vi "Top_Level_Move_Traverse.vi"(10 "Position":dbl[](array[numeric])=[0.0, 0.0, 0.0] format="%.2f", 11 "Mode":T1) -> (0 "Error String":string, 3 "Trav Position achieved":dbl[](array[numeric]) format="%.2f")   [LabVIEW 2012]
uses:
  Anemometry Sub Vis/Gen Trav/Trav_mode.ctl
  Anemometry Sub Vis/Controls/User_Specific_mode.ctl
  Anemometry Sub Vis/Globals/Trav_pos_global.vi
panel:
  out "Model       Roll      Pitch       Yaw (deg)":dbl[](array[numeric]) format="%#.2f"
  in  "Route Checking?":bool
  in  "Traverse name":string
  # "X                Y                   Z"
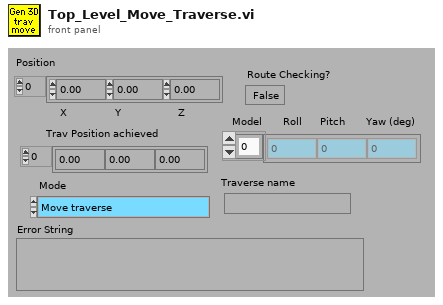
[diagram p1: front panel]
types:
  T1 = typedef "Trav_mode.ctl" = enum16{"Move traverse", "Read traverse position", "Teach Position"}
  T2 = typedef "User_Specific_mode.ctl" = enum16{"Check VI only", "Run VI"}
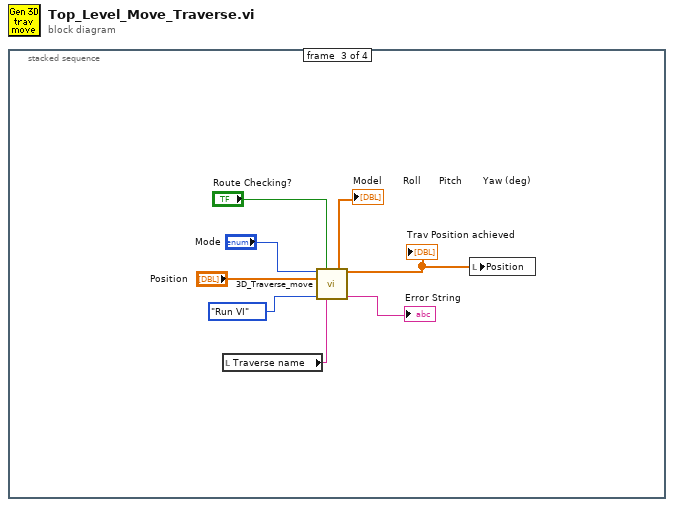
[diagram p0: block diagram]
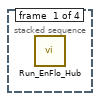
[diagram p2: hidden frame]
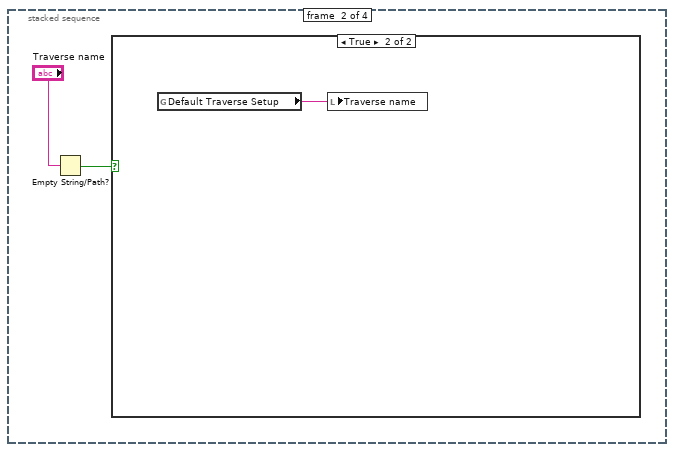
[diagram p3: hidden frame]
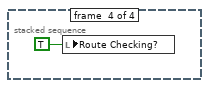
[diagram p5: hidden frame]
diagram:
  n1 = stacked-sequence {
    frame #0 {
      n2 = call "Run_EnFlo_Hub.vi"() -> ()  [unwired: 8 in]
    }
    frame #1 {
      n3 = Empty String/Path?(string/path="Traverse name") -> (empty?=w1:bool)
      n4 = case shown="True" w1 {
        frame False {
        }
        frame True {
          n5 = global read "Trav_pos_global.vi" "Default Traverse Setup"() -> (w3:string)
          n6 = local write "Traverse name"(w3) -> ()
        }
      }
    }
    frame #2 {
      n7 = local read "Traverse name"() -> (w5:string)
      n8 = call "3D_Traverse_move.vi"("Mode"="Mode", "Route Checking?"="Route Checking?", "Position"="Position", "Simulate/Run"=User_Specific_mode."Run VI", "Traverse name"=w5) -> ("Model  Roll        Pitch       Yaw (deg)"=→"Model       Roll      Pitch       Yaw (deg)":dbl[], "Trav Position achieved"=w4:dbl[], "Error String"=→"Error String":string)  [unwired: 8 in]
      "Trav Position achieved" <- w4
      n9 = local write "Position"(w4) -> ()
    }
    frame #3 {
      n10 = local write "Route Checking?"(TRUE ("Route Checking?")) -> ()
    }
  }
